vi "FA Bending Profile View.vi"() -> ()   [LabVIEW 2016, in "M1M3SupportEUI_Views.lvlib"]
uses:
  M1M3SupportEUI_Views.lvlib
  Model/Model.lvclass
  M1M3 Support Events/M1M3 Support Events.lvclass/M1M3 Support Events.ctl
  SALLV_m1m3/DataTypes/command_RunMirrorForceProfile.ctl
  SALLV_m1m3/DataTypes/command_AbortProfile.ctl
  SALLV_m1m3/DataTypes/command_ApplyAberrationForcesByBendingModes.ctl
  SALLV_m1m3/DataTypes/command_ClearAberrationForces.ctl
  SALLV_m1m3/DataTypes/command_ApplyActiveOpticForcesByBendingModes.ctl
  SALLV_m1m3/DataTypes/command_ClearActiveOpticForces.ctl
  <vilib>/Utility/file.llb/Read Delimited Spreadsheet (DBL).vi
  M1M3 Support Events/M1M3 Support Events.lvclass
  EUI Events/EUI Events.lvclass
  SALLV_m1m3/SALLV_m1m3.lvlib
panel:
  out "CSVFileArray":sgl[][](array[numeric])
  out "MirrorProfileTable":string[][](table)
  in  "UploadCSVFileButton":bool
  in  "ClearActiveOpticsButton":bool
  in  "ApplyActiveOpticsByBendingModesButton":bool
  in  "ClearAberrationButton":bool
  in  "ApplyAberrationByBendingModesButton":bool
  in  "BM21":sgl
  in  "BM20":sgl
  in  "BM22":sgl
  in  "BM11":sgl
  in  "BM10":sgl
  in  "BM19":sgl
  in  "BM18":sgl
  in  "BM17":sgl
  in  "BM16":sgl
  in  "BM15":sgl
  in  "BM14":sgl
  in  "BM13":sgl
  in  "BM12":sgl
  in  "BM1":sgl
  in  "BM9":sgl
  in  "BM8":sgl
  in  "BM7":sgl
  in  "BM6":sgl
  in  "BM5":sgl
  in  "BM4":sgl
  in  "BM3":sgl
  in  "BM2":sgl
  in  "AbortProfileButton":bool
  in  "RunMirrorForceProfileButton":bool
  in  "Model in":refnum<class "Model.lvclass">
  # "Force Actuator\nApply/Clear Bending Modes\nRun/Abort Mirror Force Profile"
  # "Bending Modes"
  # "0"
  # "1"
  # "2"
  # "3"
  # "4"
  # "5"
  # "6"
  # "7"
  # "8"
  # "9"
  # "00"
  # "10"
  # "Force Profile"
  # "20"
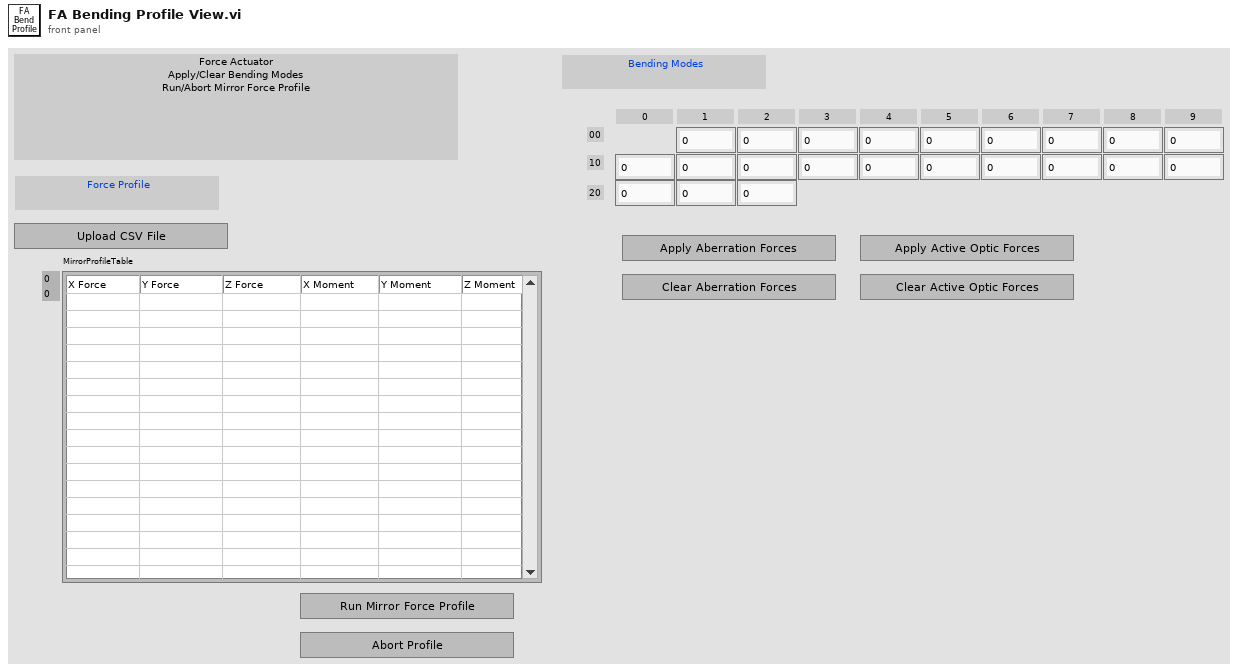
[diagram p1: front panel]
types:
  T1 = typedef "M1M3SupportEUI_TypeDefs.lvlib/M1M3 Support Events.ctl" = cluster{"Inclinometer  Data":refnum<user-event>, "IMS Data":refnum<user-event>, "SAL Connected":refnum<user-event>, "Accelerometer Data":refnum<user-event>, "OuterLoop Data":refnum<user-event>, "ErrorCode Event":refnum<user-event>, "InterlockStatus Event":refnum<user-event>, "InterlockWarning Event":refnum<user-event>, "Gyro Data":refnum<user-event>, "HP Actuator Info Event":refnum<user-event>, " FA Info Event":refnum<user-event>, "HP Monitor Info Event":refnum<user-event>, "FA Data":refnum<user-event>, "HP Actuator data":refnum<user-event>, "HP Monitor data":refnum<user-event>, "Air Supply Status Event":refnum<user-event>, "Air Supply Warning Event":refnum<user-event>, "Power Data":refnum<user-event>, "PID Data":refnum<user-event>, "PID Info Event":refnum<user-event>, "Power Status Event":refnum<user-event>, "Power Supply Status Event":refnum<user-event>, "Power Warning Event":refnum<user-event>, "Summary State Event":refnum<user-event>, "Detailed State Event":refnum<user-event>, "FA Force Warning Event":refnum<user-event>, "FA Warning Event":refnum<user-event>, "FA State Event":refnum<user-event>, "Applied AberrationForces Event":refnum<user-event>, "Applied Acceleration Forcces Event":refnum<user-event>, "Applied Azimuth Forces Event":refnum<user-event>, "Applied Active Optic Forces Event":refnum<user-event>, "Applied Balance Forces Event":refnum<user-event>, "Applied Cylinder Forces Event":refnum<user-event>, "Applied Elevation Forces Event":refnum<user-event>, "Applied Forces Event":refnum<user-event>, "Applied Offset Forces Event":refnum<user-event>, "Applied Static Forces Event":refnum<user-event>, "Applied Thermal Forces Event":refnum<user-event>, "Applied Velocity Forces Event":refnum<user-event>, "Rejected Aberration Force Event":refnum<user-event>, "Rejected Acceleration Forces Event":refnum<user-event>, "Rejected Active Optic Forces Event":refnum<user-event>, "Rejected Azimuth Forces Event":refnum<user-event>, "Rejected Balance Forces Event":refnum<user-event>, "Rejected Cylinder Forces Event":refnum<user-event>, "Rejected Elevation Forces Event":refnum<user-event>, "Rejected Forces Event":refnum<user-event>, "Rejected Offset Forces Event":refnum<user-event>, "Rejected Static Forces Event":refnum<user-event>, "Rejected Thermal Forces Event":refnum<user-event>, "Rejected Velocity Forces Event":refnum<user-event>, "Command Rejection Event":refnum<user-event>, "Setting Verions Event":refnum<user-event>, "Settings Applied Event":refnum<user-event>, "HP Actuator State Event":refnum<user-event>, "HP Actuator Warning Event":refnum<user-event>, "HP Monitor State Event":refnum<user-event>, "HP Monitor Warning Event":refnum<user-event>, "Accelerometer Warning Event":refnum<user-event>, "Applied Settings Match Start Event":refnum<user-event>, "Cell Light Status Event ":refnum<user-event>, "Cell Light Warning Event":refnum<user-event>, "Displacement Sensor Warning Event":refnum<user-event>, "Force Setpoint Warning Event":refnum<user-event>, "Gyro Warning Event ":refnum<user-event>, "ILC Warning Event ":refnum<user-event>, "Inclinometer Sensor Warning Event ":refnum<user-event>}
  T2 = enum16{"", "DetailedState_DetailedStates_DisabledState", "DetailedState_DetailedStates_EnabledState", "DetailedState_DetailedStates_FaultState", "DetailedState_DetailedStates_OfflineState", "DetailedState_DetailedStates_StandbyState", "DetailedState_DetailedStates_ParkedState", "DetailedState_DetailedStates_RaisingState", "DetailedState_DetailedStates_ActiveState", "DetailedState_DetailedStates_LoweringState", "DetailedState_DetailedStates_EngineeringState", "DetailedState_DetailedStates_ParkedEngineeringState", "DetailedState_DetailedStates_RaisingEngineeringState", "DetailedState_DetailedStates_ActiveEngineeringState", "DetailedState_DetailedStates_LoweringEngineeringState", "DetailedState_DetailedStates_LoweringFaultState", "DetailedState_DetailedStates_ProfileHardpointCorrectionState"}
  T3 = typedef "SALLV_m1m3.lvlib/command_RunMirrorForceProfile.ctl" = cluster{"XForce[1000]":sgl[], "YForce[1000]":sgl[], "ZForce[1000]":sgl[], "XMoment[1000]":sgl[], "YMoment[1000]":sgl[], "ZMoment[1000]":sgl[]}
  T4 = typedef "SALLV_m1m3.lvlib/command_AbortProfile.ctl" = cluster{"AbortProfile":bool}
  T5 = typedef "SALLV_m1m3.lvlib/command_ApplyAberrationForcesByBendingModes.ctl" = cluster{"Coefficients[22]":sgl[]}
  T6 = typedef "SALLV_m1m3.lvlib/command_ClearAberrationForces.ctl" = cluster{"ClearAberrationForces":bool}
  T7 = typedef "SALLV_m1m3.lvlib/command_ApplyActiveOpticForcesByBendingModes.ctl" = cluster{"Coefficients[22]":sgl[]}
  T8 = typedef "SALLV_m1m3.lvlib/command_ClearActiveOpticForces.ctl" = cluster{"ClearActiveOpticForces":bool}
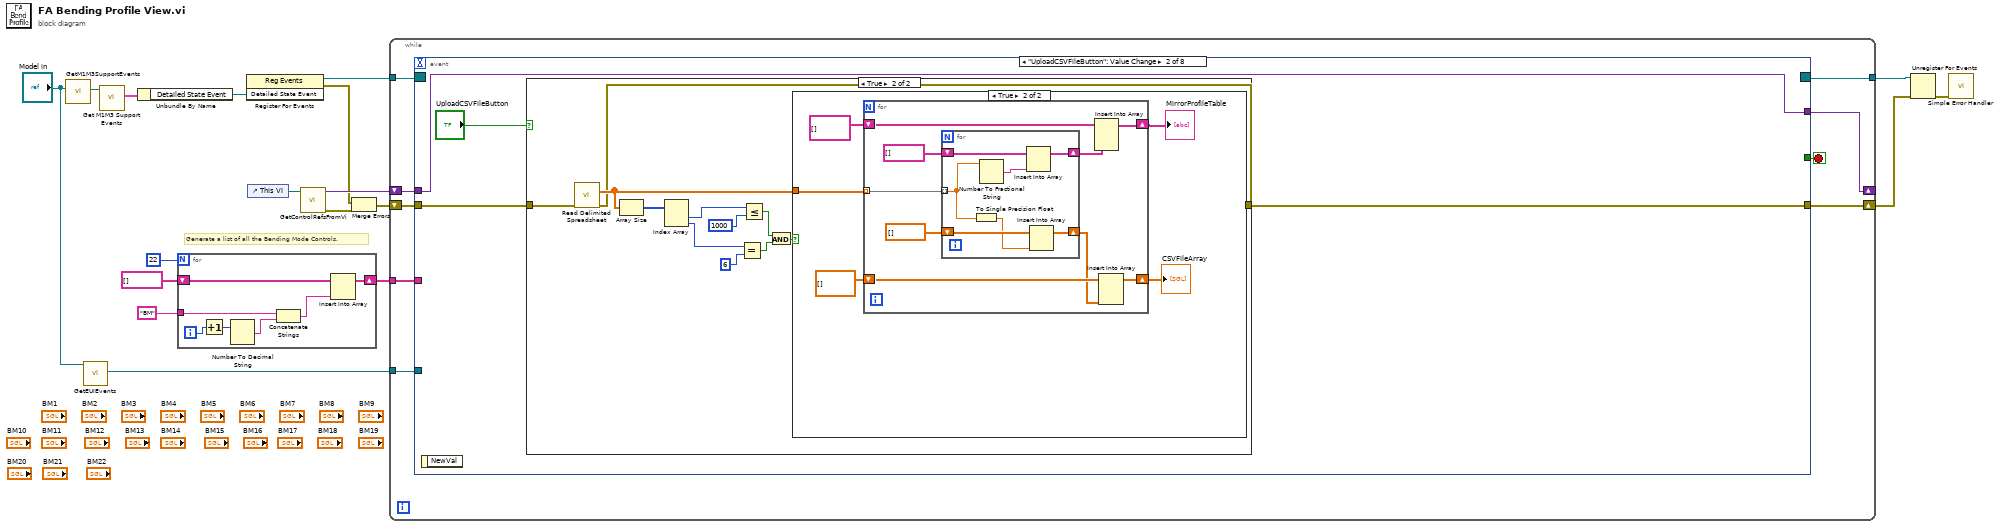
[diagram p0: block diagram]
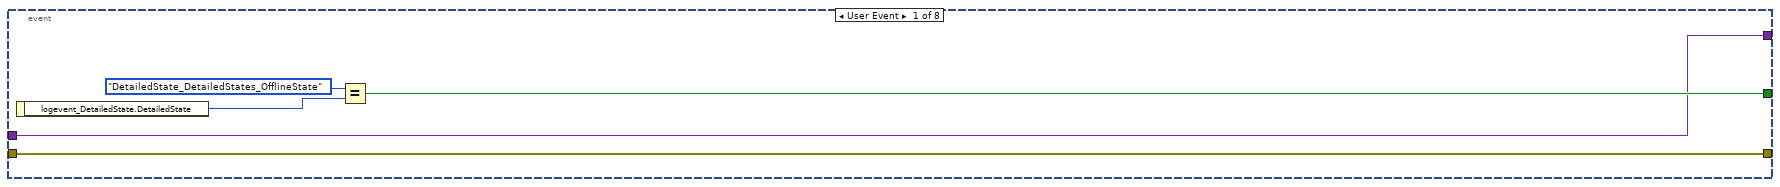
[diagram p2: hidden frame]
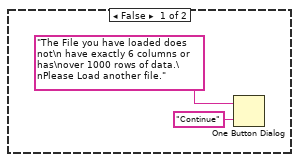
[diagram p4: hidden frame]
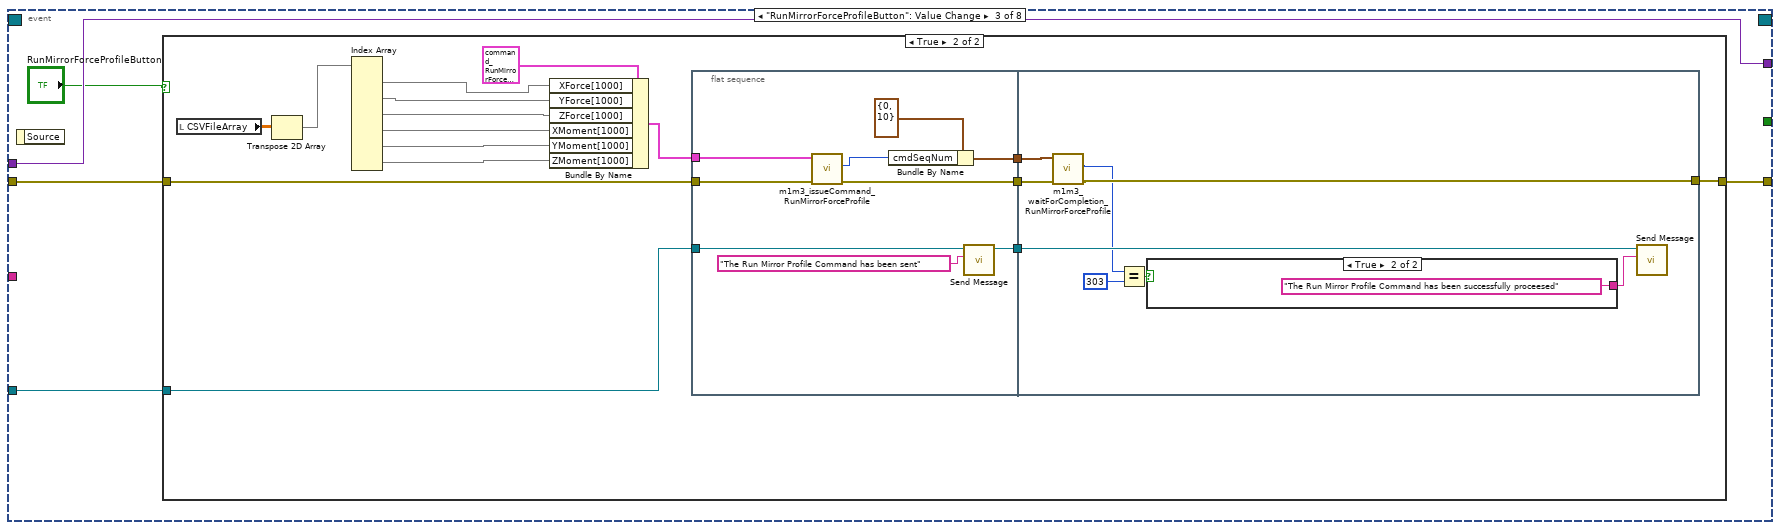
[diagram p5: hidden frame]
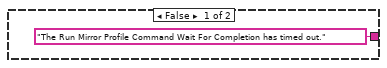
[diagram p7: hidden frame]
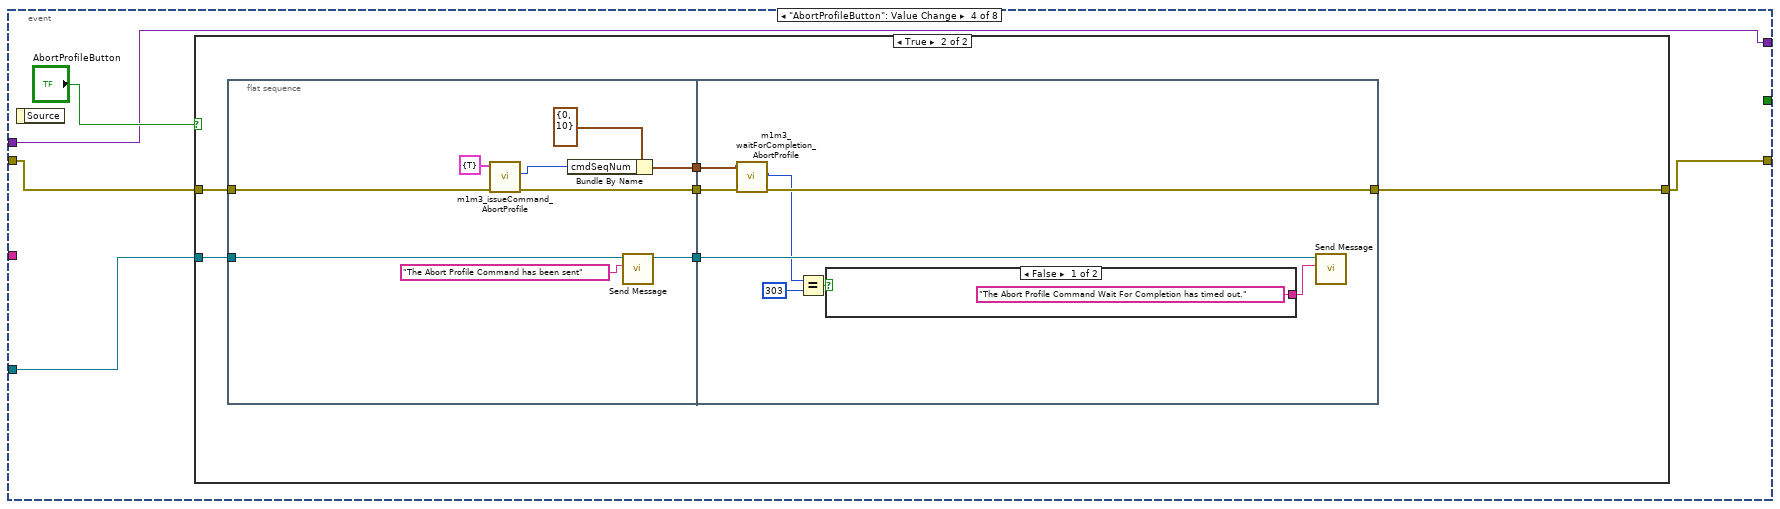
[diagram p8: hidden frame]
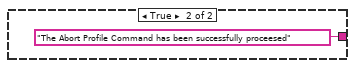
[diagram p10: hidden frame]
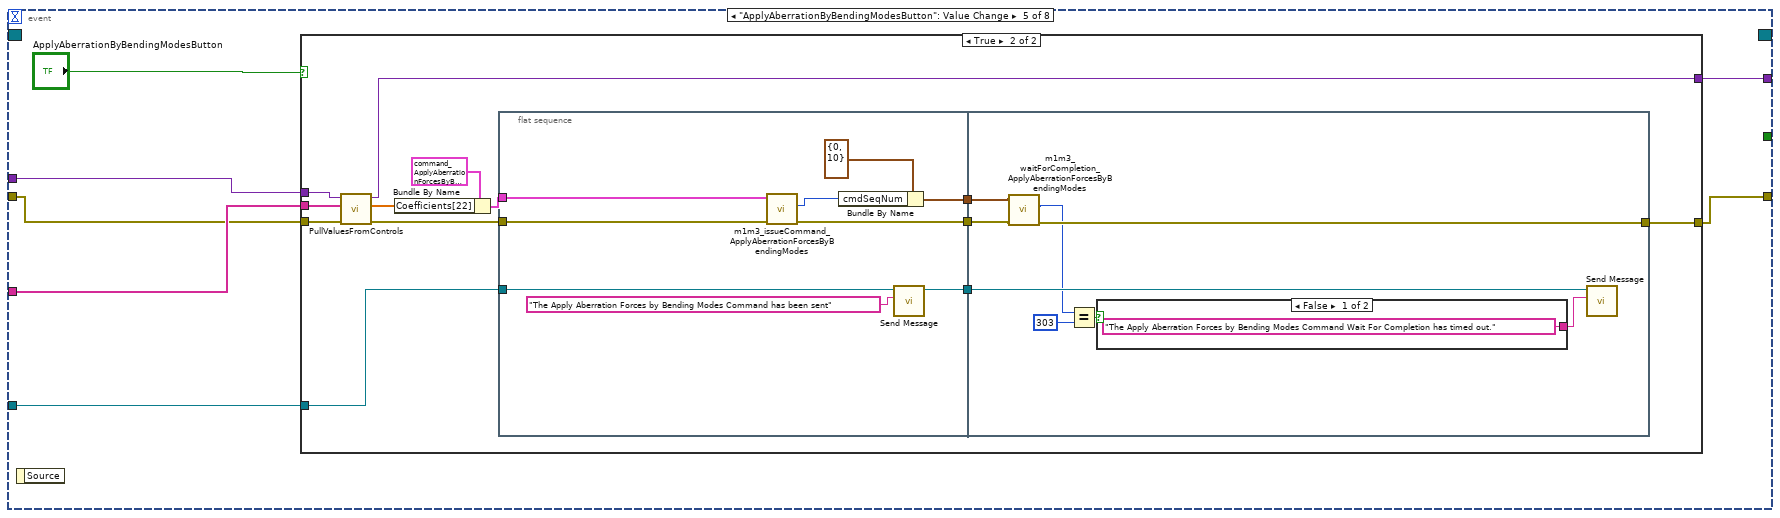
[diagram p11: hidden frame]
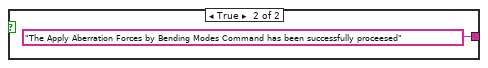
[diagram p13: hidden frame]
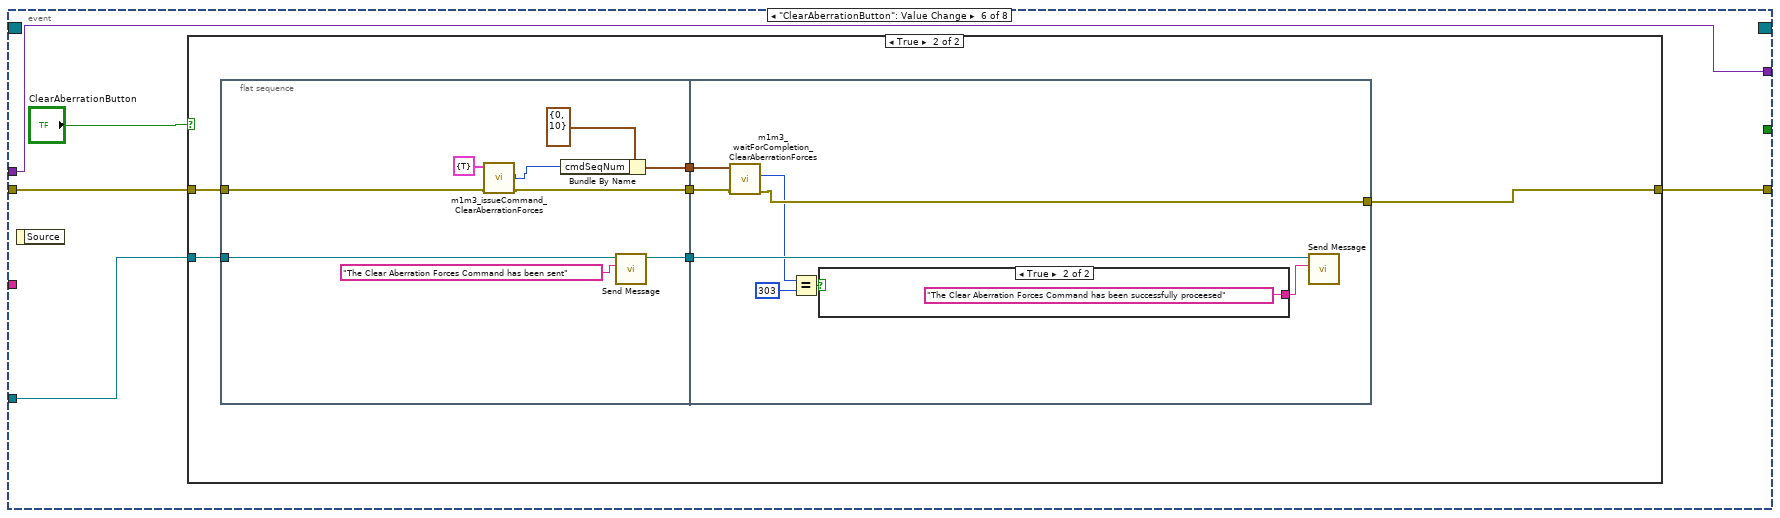
[diagram p14: hidden frame]
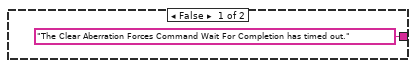
[diagram p16: hidden frame]
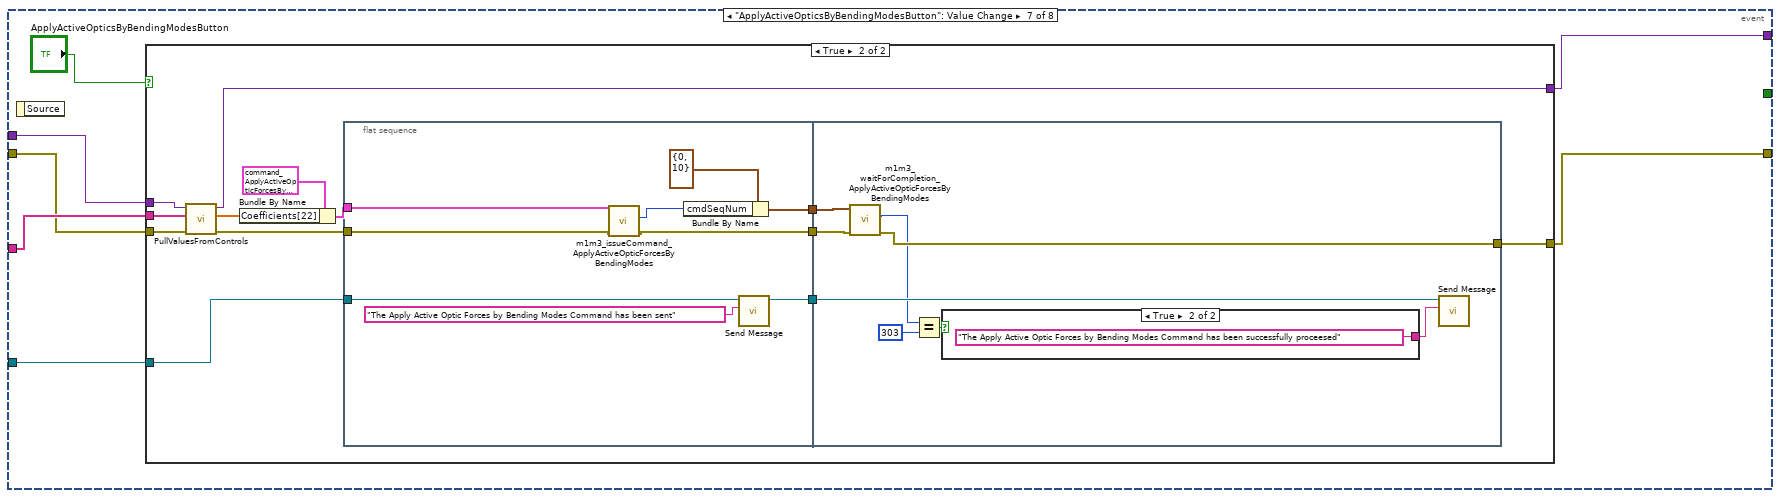
[diagram p17: hidden frame]
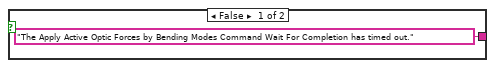
[diagram p19: hidden frame]
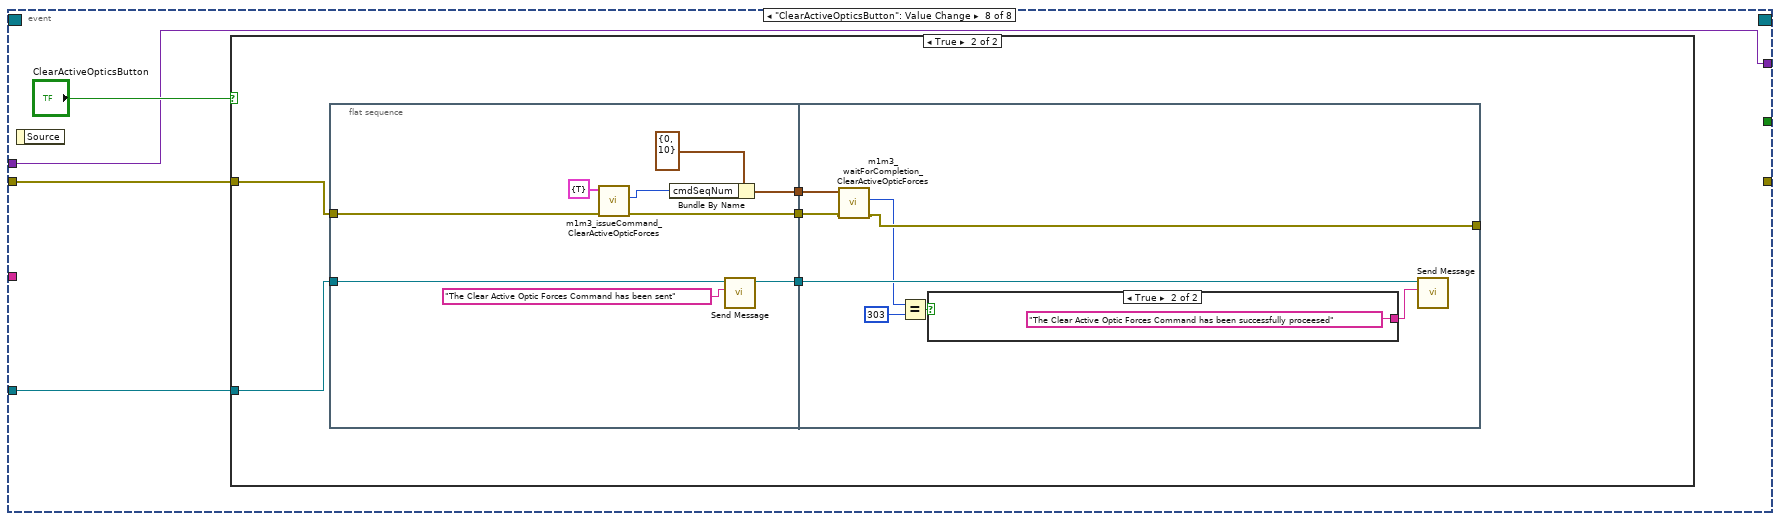
[diagram p20: hidden frame]
diagram:
  # "Generate a list of all the Bending Mode Controls."
  n1 = call "GetM1M3SupportEvents.vi"("Model in"="Model in") -> ("M1M3 Support Events out"=w17:refnum<class "M1M3 Support Events.lvclass">)  [unwired: 8 in, 2 out]
  n2 = call "GetEUIEvents.vi"("Model in"="Model in") -> ("EUI Events out"=w5:refnum<class "EUI Events.lvclass">)  [unwired: 8 in, 2 out]
  n3 = call "Get M1M3 Support Events.vi"("M1M3 Support Events in"=w17) -> ("M1M3 Support Events"=w18:T1)  [unwired: 9 in, 1 out]
  n4 = Unbundle By Name(w18) -> ("Detailed State Event"=w16:refnum<user-event>)
  n5 = for {
    N: 22 -> [_]
    shift-right: [w24] -> w11
    shift-left: string[] [] -> [w25]
    tunnel: "BM" -> [w23]
    i -> [w19]
    n6 = Increment(x=w19) -> (x+1=w20:i32)
    n7 = Number To Decimal String(number=w20) -> (decimal integer string=w22:string)  [unwired: 1 in]
    n8 = Concatenate Strings(w23, w22) -> (w21:string)
    n9 = Insert Into Array(array=w25, new element=w21) -> (w24:string[])  [unwired: 1 in]
  }
  n10 = register-events(w16) -> (reference out=w15:refnum<event-registration>, error out=w9:errorcluster)  [unwired: 2 in]
  n11 = control-ref of="This VI"() -> (w1:refnum<vi>)
  n12 = call "GetControlRefsFromVi.vi"("VI Refnum"=w1) -> ("error out"=w8:errorcluster, "Variant"=w10:variant)  [unwired: 9 in]
  n13 = Merge Errors(w9, w8) -> (w7:errorcluster)
  n14 = while {
    tunnel: w15 -> [w34]
    tunnel: w11 -> [w32]
    shift-right: [w28] -> w3
    shift-left: w7 -> [w30]
    tunnel: w5 -> [w29]
    shift-right: [w27] -> _
    shift-left: w10 -> [w31]
    tunnel: [w26] -> w4
    stop <- w33 stop-if-true
    n15 = event shown="[1] \"UploadCSVFileButton\": Value Change" {
      selector: w34 -> [_ _ _ _ _ _ _ _]
      dyn-events: [_ _ _ _ _ _ _ _] -> w26
      timeout: _ -> [_ _ _ _ _ _ _ _]
      tunnel: [w37 _ _ _ _ _ _ _] -> w33
      tunnel: w32 -> [_ _ _ _ w155 _ w227 _]
      tunnel: w31 -> [w36 w41 w83 w121 w156 w192 w228 w266]
      tunnel: w30 -> [w35 w42 w81 w122 w154 w196 w226 w265]
      tunnel: w29 -> [_ _ w79 w123 w153 w194 w225 w264]
      tunnel: [w35 w40 w80 w120 w152 w193 w224 _] -> w28
      tunnel: [w36 w41 w83 w121 w151 w192 w223 w266] -> w27
      event User Event {
        n16 = event-data() -> ("logevent_DetailedState.DetailedState"=w39:T2)  [unwired: 1 in]
        n17 = Equal?(x=T2."DetailedState_DetailedStates_OfflineState", y=w39) -> (x = y?=w37:bool)
      }
      event "UploadCSVFileButton": Value Change {
        n18 = event-data() -> ()  [unwired: 1 in, 1 out]
        n19 = case shown="True" "UploadCSVFileButton" {
          tunnel: w42 -> [w44 w55]
          tunnel: [w44 w50] -> w40
          frame False {
          }
          frame True {
            n20 = call-poly <vilib>:"Read Delimited Spreadsheet.vi"("error in (no error)"=w55) -> ("all rows"=w54:dbl[][], "error out"=w50:errorcluster)  [unwired: 9 in, 4 out]
            n21 = Array Size(array=w54) -> (size(s)=w49:i32[])
            n22 = Index Array(array=w49) -> (element #1=w48:i32, element #2=w45:i32)  [unwired: 2 in]
            n23 = Equal?(x=w45, y=6) -> (x = y?=w46:bool)
            n24 = Less Or Equal?(x=w48, y=1000) -> (x <= y?=w47:bool)
            n25 = And(x=w47, y=w46) -> (x .and. y?=w51:bool)
            n26 = case shown="True" w51 {
              tunnel: w54 -> [_ w62]
              frame False {
                n27 = One Button Dialog(message="The File you have loaded does not\n have exactly 6 columns or has\nover 1000 rows of data.\nPlease Load another file.", button name ("OK")="Continue") -> ()  [unwired: 1 out]
              }
              frame True {
                n28 = for {
                  tunnel: w62 -> [w71] mode=indexing
                  shift-right: [w68] -> w59
                  shift-left: string[][] [] -> [w69]
                  shift-right: [w63] -> w58
                  shift-left: sgl[][] [] -> [w65]
                  n29 = for {
                    tunnel: w71 -> [w75] mode=indexing
                    shift-right: [w77] -> w67
                    shift-left: string[] [] -> [w78]
                    shift-right: [w73] -> w64
                    shift-left: sgl[] [] -> [w74]
                    n30 = To Single Precision Float(number=w75) -> (single precision float=w72:sgl)
                    n31 = Number To Fractional String(number=w75) -> (F-format string=w76:string)  [unwired: 3 in]
                    n32 = Insert Into Array(array=w78, new element=w76) -> (w77:string[])  [unwired: 1 in]
                    n33 = Insert Into Array(array=w74, new element=w72) -> (w73:sgl[])  [unwired: 1 in]
                  }
                  n34 = Insert Into Array(array=w69, new element=w67) -> (w68:string[][])  [unwired: 2 in]
                  n35 = Insert Into Array(array=w65, new element=w64) -> (w63:sgl[][])  [unwired: 2 in]
                }
                "MirrorProfileTable" <- w59
                "CSVFileArray" <- w58
              }
            }
          }
        }
      }
      event "RunMirrorForceProfileButton": Value Change {
        n36 = event-data() -> ()  [unwired: 1 in, 1 out]
        n37 = case shown="True" "RunMirrorForceProfileButton" {
          tunnel: w81 -> [w84 w93]
          tunnel: [w84 w92] -> w80
          tunnel: w79 -> [_ w96]
          frame False {
          }
          frame True {
            n38 = local read "CSVFileArray"() -> (w97:sgl[][])
            n39 = Transpose 2D Array(2D array=w97) -> (transposed array=w91:sgl[][])
            n40 = Index Array(array=w91) -> (element #1=w90:sgl[], element #2=w89:sgl[], element #3=w88:sgl[], element #4=w87:sgl[], element #5=w86:sgl[], element #6=w85:sgl[])  [unwired: 12 in]
            n41 = Bundle By Name(cluster=T3 {"XForce[1000]"=array[1000 elements], "YForce[1000]"=array[1000 elements], "ZForce[1000]"=array[1000 elements], "XMoment[1000]"=array[1000 elements], "YMoment[1000]"=array[1000 elements], "ZMoment[1000]"=array[1000 elements]} ("command_RunMirrorForceProfile"), "XForce[1000]"=w90, "YForce[1000]"=w89, "ZForce[1000]"=w88, "XMoment[1000]"=w87, "YMoment[1000]"=w86, "ZMoment[1000]"=w85) -> (w94:T3)
            n42 = flat-sequence {
              tunnel: [w108] -> w100
              tunnel: [w103] -> w99
              tunnel: [w106] -> w98
              tunnel: w96 -> [w105]
              tunnel: w94 -> [w101]
              tunnel: w93 -> [w104]
              tunnel: w100 -> [w114]
              tunnel: w99 -> [w112]
              tunnel: [w111] -> w92
              tunnel: w98 -> [w113]
              frame #0 {
                n43 = call "m1m3_issueCommand_RunMirrorForceProfile.vi"("error in (no error)"=w104, "command_RunMirrorForceProfile_Ctl"=w101) -> ("error out"=w103:errorcluster, "function return"=w102:i32)  [unwired: 7 in, 1 out]
                n44 = Bundle By Name(cluster=cluster{"cmdSeqNum":i32, "timeout":u32} {"cmdSeqNum"=0, "timeout"=10} ("waitComplete_Ctl"), "cmdSeqNum"=w102) -> (w106:cluster{"cmdSeqNum":i32, "timeout":u32})
                n45 = call "Send Message.vi"("Message"="The Run Mirror Profile Command has been sent", "EUI Events in"=w105) -> ("EUI Events out"=w108:refnum<class "EUI Events.lvclass">)  [unwired: 8 in, 1 out]
              }
              frame #1 {
                n46 = call "m1m3_waitForCompletion_RunMirrorForceProfile.vi"("error in (no error)"=w112, "waitComplete_Ctl"=w113) -> ("error out"=w111:errorcluster, "function return"=w110:i32)  [unwired: 7 in, 1 out]
                n47 = Equal?(x=w110, y=303) -> (x = y?=w116:bool)
                n48 = case shown="True" w116 {
                  tunnel: ["The Run Mirror Profile Command Wait For Completion has timed out." ("Message") "The Run Mirror Profile Command has been successfully proceesed" ("Message")] -> w117
                  frame False {
                  }
                  frame True {
                  }
                }
                n49 = call "Send Message.vi"("Message"=w117, "EUI Events in"=w114) -> ()  [unwired: 8 in, 2 out]
              }
            }
          }
        }
      }
      event "AbortProfileButton": Value Change {
        n50 = event-data() -> ()  [unwired: 1 in, 1 out]
        n51 = case shown="True" "AbortProfileButton" {
          tunnel: w122 -> [w125 w128]
          tunnel: w123 -> [_ w127]
          tunnel: [w125 w126] -> w120
          frame False {
          }
          frame True {
            n52 = flat-sequence {
              tunnel: [w139] -> w131
              tunnel: w128 -> [w135]
              tunnel: [w132] -> w130
              tunnel: [w137] -> w129
              tunnel: w127 -> [w136]
              tunnel: w131 -> [w145]
              tunnel: w130 -> [w143]
              tunnel: [w142] -> w126
              tunnel: w129 -> [w144]
              frame #0 {
                n53 = call "m1m3_issueCommand_AbortProfile.vi"("error in (no error)"=w135, "command_AbortProfile_Ctl"=T4 {"AbortProfile"=TRUE}) -> ("error out"=w132:errorcluster, "function return"=w133:i32)  [unwired: 7 in, 1 out]
                n54 = Bundle By Name(cluster=cluster{"cmdSeqNum":i32, "timeout":u32} {"cmdSeqNum"=0, "timeout"=10} ("waitComplete_Ctl"), "cmdSeqNum"=w133) -> (w137:cluster{"cmdSeqNum":i32, "timeout":u32})
                n55 = call "Send Message.vi"("Message"="The Abort Profile Command has been sent", "EUI Events in"=w136) -> ("EUI Events out"=w139:refnum<class "EUI Events.lvclass">)  [unwired: 8 in, 1 out]
              }
              frame #1 {
                n56 = call "m1m3_waitForCompletion_AbortProfile.vi"("error in (no error)"=w143, "waitComplete_Ctl"=w144) -> ("error out"=w142:errorcluster, "function return"=w141:i32)  [unwired: 7 in, 1 out]
                n57 = Equal?(x=w141, y=303) -> (x = y?=w147:bool)
                n58 = case shown="False" w147 {
                  tunnel: ["The Abort Profile Command Wait For Completion has timed out." ("Message") "The Abort Profile Command has been successfully proceesed" ("Message")] -> w148
                  frame False {
                  }
                  frame True {
                  }
                }
                n59 = call "Send Message.vi"("Message"=w148, "EUI Events in"=w145) -> ()  [unwired: 8 in, 2 out]
              }
            }
          }
        }
      }
      event "ApplyAberrationByBendingModesButton": Value Change {
        n60 = event-data() -> ()  [unwired: 1 in, 1 out]
        n61 = case shown="True" "ApplyAberrationByBendingModesButton" {
          tunnel: w156 -> [w158 w170]
          tunnel: w154 -> [w159 w169]
          tunnel: [w159 w166] -> w152
          tunnel: [w158 w163] -> w151
          tunnel: w155 -> [_ w162]
          tunnel: w153 -> [_ w161]
          frame False {
          }
          frame True {
            n62 = call "PullValuesFromControls.vi"("error in (no error)"=w169, "ControlNameArray"=w162, "Variant In"=w170) -> ("error out"=w168:errorcluster, "ControlValuesArray"=w171:sgl[], "Variant out"=w163:variant)  [unwired: 6 in]
            n63 = Bundle By Name(cluster=T5 {"Coefficients[22]"=[0.0, 0.0, 0.0, 0.0, 0.0, 0.0, 0.0, 0.0, 0.0, 0.0, 0.0, 0.0, 0.0, 0.0, 0.0, 0.0, 0.0, 0.0, 0.0, 0.0, 0.0, 0.0]} ("command_ApplyAberrationForcesByBendingModes"), "Coefficients[22]"=w171) -> (w165:T5)
            n64 = flat-sequence {
              tunnel: [w180] -> w172
              tunnel: w168 -> [w175]
              tunnel: [w173] -> w167
              tunnel: w165 -> [w176]
              tunnel: [w178] -> w164
              tunnel: w161 -> [w177]
              tunnel: w172 -> [w186]
              tunnel: w167 -> [w184]
              tunnel: [w183] -> w166
              tunnel: w164 -> [w185]
              frame #0 {
                n65 = call "m1m3_issueCommand_ApplyAberrationForcesByBendingModes.vi"("error in (no error)"=w175, "command_ApplyAberrationForcesByBendingModes_Ctl"=w176) -> ("error out"=w173:errorcluster, "function return"=w174:i32)  [unwired: 7 in, 1 out]
                n66 = Bundle By Name(cluster=cluster{"cmdSeqNum":i32, "timeout":u32} {"cmdSeqNum"=0, "timeout"=10} ("waitComplete_Ctl"), "cmdSeqNum"=w174) -> (w178:cluster{"cmdSeqNum":i32, "timeout":u32})
                n67 = call "Send Message.vi"("Message"="The Apply Aberration Forces by Bending Modes Command has been sent", "EUI Events in"=w177) -> ("EUI Events out"=w180:refnum<class "EUI Events.lvclass">)  [unwired: 8 in, 1 out]
              }
              frame #1 {
                n68 = call "m1m3_waitForCompletion_ApplyAberrationForcesByBendingModes.vi"("error in (no error)"=w184, "waitComplete_Ctl"=w185) -> ("error out"=w183:errorcluster, "function return"=w182:i32)  [unwired: 7 in, 1 out]
                n69 = Equal?(x=w182, y=303) -> (x = y?=w188:bool)
                n70 = case shown="False" w188 {
                  tunnel: ["The Apply Aberration Forces by Bending Modes Command Wait For Completion has timed out." ("Message") "The Apply Aberration Forces by Bending Modes Command has been successfully proceesed" ("Message")] -> w189
                  frame False {
                  }
                  frame True {
                  }
                }
                n71 = call "Send Message.vi"("Message"=w189, "EUI Events in"=w186) -> ()  [unwired: 8 in, 2 out]
              }
            }
          }
        }
      }
      event "ClearAberrationButton": Value Change {
        n72 = event-data() -> ()  [unwired: 1 in, 1 out]
        n73 = case shown="True" "ClearAberrationButton" {
          tunnel: w196 -> [w197 w200]
          tunnel: w194 -> [_ w199]
          tunnel: [w197 w198] -> w193
          frame False {
          }
          frame True {
            n74 = flat-sequence {
              tunnel: [w211] -> w203
              tunnel: w200 -> [w207]
              tunnel: [w206] -> w202
              tunnel: [w209] -> w201
              tunnel: w199 -> [w208]
              tunnel: w203 -> [w217]
              tunnel: w202 -> [w215]
              tunnel: [w214] -> w198
              tunnel: w201 -> [w216]
              frame #0 {
                n75 = call "m1m3_issueCommand_ClearAberrationForces.vi"("error in (no error)"=w207, "command_ClearAberrationForces_Ctl"=T6 {"ClearAberrationForces"=TRUE}) -> ("error out"=w206:errorcluster, "function return"=w205:i32)  [unwired: 7 in, 1 out]
                n76 = Bundle By Name(cluster=cluster{"cmdSeqNum":i32, "timeout":u32} {"cmdSeqNum"=0, "timeout"=10} ("waitComplete_Ctl"), "cmdSeqNum"=w205) -> (w209:cluster{"cmdSeqNum":i32, "timeout":u32})
                n77 = call "Send Message.vi"("Message"="The Clear Aberration Forces Command has been sent", "EUI Events in"=w208) -> ("EUI Events out"=w211:refnum<class "EUI Events.lvclass">)  [unwired: 8 in, 1 out]
              }
              frame #1 {
                n78 = call "m1m3_waitForCompletion_ClearAberrationForces.vi"("error in (no error)"=w215, "waitComplete_Ctl"=w216) -> ("error out"=w214:errorcluster, "function return"=w213:i32)  [unwired: 7 in, 1 out]
                n79 = Equal?(x=w213, y=303) -> (x = y?=w219:bool)
                n80 = case shown="True" w219 {
                  tunnel: ["The Clear Aberration Forces Command Wait For Completion has timed out." ("Message") "The Clear Aberration Forces Command has been successfully proceesed" ("Message")] -> w220
                  frame False {
                  }
                  frame True {
                  }
                }
                n81 = call "Send Message.vi"("Message"=w220, "EUI Events in"=w217) -> ()  [unwired: 8 in, 2 out]
              }
            }
          }
        }
      }
      event "ApplyActiveOpticsByBendingModesButton": Value Change {
        n82 = event-data() -> ()  [unwired: 1 in, 1 out]
        n83 = case shown="True" "ApplyActiveOpticsByBendingModesButton" {
          tunnel: w228 -> [w230 w242]
          tunnel: w226 -> [w231 w241]
          tunnel: [w231 w238] -> w224
          tunnel: [w230 w235] -> w223
          tunnel: w227 -> [_ w234]
          tunnel: w225 -> [_ w233]
          frame False {
          }
          frame True {
            n84 = call "PullValuesFromControls.vi"("error in (no error)"=w241, "ControlNameArray"=w234, "Variant In"=w242) -> ("error out"=w240:errorcluster, "ControlValuesArray"=w243:sgl[], "Variant out"=w235:variant)  [unwired: 6 in]
            n85 = Bundle By Name(cluster=T7 {"Coefficients[22]"=[0.0, 0.0, 0.0, 0.0, 0.0, 0.0, 0.0, 0.0, 0.0, 0.0, 0.0, 0.0, 0.0, 0.0, 0.0, 0.0, 0.0, 0.0, 0.0, 0.0, 0.0, 0.0]} ("command_ApplyActiveOpticForcesByBendingModes"), "Coefficients[22]"=w243) -> (w237:T7)
            n86 = flat-sequence {
              tunnel: [w252] -> w244
              tunnel: w240 -> [w246]
              tunnel: [w248] -> w239
              tunnel: w237 -> [w245]
              tunnel: [w250] -> w236
              tunnel: w233 -> [w249]
              tunnel: w244 -> [w258]
              tunnel: w239 -> [w254]
              tunnel: [w256] -> w238
              tunnel: w236 -> [w257]
              frame #0 {
                n87 = call "m1m3_issueCommand_ApplyActiveOpticForcesByBendingModes.vi"("error in (no error)"=w246, "command_ApplyActiveOpticForcesByBendingModes_Ctl"=w245) -> ("error out"=w248:errorcluster, "function return"=w247:i32)  [unwired: 7 in, 1 out]
                n88 = Bundle By Name(cluster=cluster{"cmdSeqNum":i32, "timeout":u32} {"cmdSeqNum"=0, "timeout"=10} ("waitComplete_Ctl"), "cmdSeqNum"=w247) -> (w250:cluster{"cmdSeqNum":i32, "timeout":u32})
                n89 = call "Send Message.vi"("Message"="The Apply Active Optic Forces by Bending Modes Command has been sent", "EUI Events in"=w249) -> ("EUI Events out"=w252:refnum<class "EUI Events.lvclass">)  [unwired: 8 in, 1 out]
              }
              frame #1 {
                n90 = call "m1m3_waitForCompletion_ApplyActiveOpticForcesByBendingModes.vi"("error in (no error)"=w254, "waitComplete_Ctl"=w257) -> ("error out"=w256:errorcluster, "function return"=w255:i32)  [unwired: 7 in, 1 out]
                n91 = Equal?(x=w255, y=303) -> (x = y?=w260:bool)
                n92 = case shown="True" w260 {
                  tunnel: ["The Apply Active Optic Forces by Bending Modes Command Wait For Completion has timed out." ("Message") "The Apply Active Optic Forces by Bending Modes Command has been successfully proceesed" ("Message")] -> w261
                  frame False {
                  }
                  frame True {
                  }
                }
                n93 = call "Send Message.vi"("Message"=w261, "EUI Events in"=w258) -> ()  [unwired: 8 in, 2 out]
              }
            }
          }
        }
      }
      event "ClearActiveOpticsButton": Value Change {
        n94 = event-data() -> ()  [unwired: 1 in, 1 out]
        n95 = case shown="True" "ClearActiveOpticsButton" {
          tunnel: w265 -> [_ w269]
          tunnel: w264 -> [_ w268]
          frame False {
          }
          frame True {
            n96 = flat-sequence {
              tunnel: [w280] -> w272
              tunnel: w269 -> [w276]
              tunnel: [w275] -> w271
              tunnel: [w278] -> w270
              tunnel: w268 -> [w277]
              tunnel: w272 -> [w286]
              tunnel: w271 -> [w284]
              tunnel: [w283] -> _
              tunnel: w270 -> [w285]
              frame #0 {
                n97 = call "m1m3_issueCommand_ClearActiveOpticForces.vi"("error in (no error)"=w276, "command_ClearActiveOpticForces_Ctl"=T8 {"ClearActiveOpticForces"=TRUE}) -> ("error out"=w275:errorcluster, "function return"=w274:i32)  [unwired: 7 in, 1 out]
                n98 = Bundle By Name(cluster=cluster{"cmdSeqNum":i32, "timeout":u32} {"cmdSeqNum"=0, "timeout"=10} ("waitComplete_Ctl"), "cmdSeqNum"=w274) -> (w278:cluster{"cmdSeqNum":i32, "timeout":u32})
                n99 = call "Send Message.vi"("Message"="The Clear Active Optic Forces Command has been sent", "EUI Events in"=w277) -> ("EUI Events out"=w280:refnum<class "EUI Events.lvclass">)  [unwired: 8 in, 1 out]
              }
              frame #1 {
                n100 = call "m1m3_waitForCompletion_ClearActiveOpticForces.vi"("error in (no error)"=w284, "waitComplete_Ctl"=w285) -> ("error out"=w283:errorcluster, "function return"=w282:i32)  [unwired: 7 in, 1 out]
                n101 = Equal?(x=w282, y=303) -> (x = y?=w288:bool)
                n102 = case shown="True" w288 {
                  tunnel: ["The Clear Active Optic Forces Command Wait For Completion has timed out." ("Message") "The Clear Active Optic Forces Command has been successfully proceesed" ("Message")] -> w289
                  frame False {
                  }
                  frame True {
                  }
                }
                n103 = call "Send Message.vi"("Message"=w289, "EUI Events in"=w286) -> ()  [unwired: 8 in, 2 out]
              }
            }
          }
        }
      }
    }
  }
  n104 = Unregister For Events(event registration refnum=w4, error in=w3) -> (error out=w2:errorcluster)
  n105 = call <vilib>:"Simple Error Handler.vi"("error in (no error)"=w2) -> ()  [unwired: 4 in, 5 out]
